vi "Manage Frame.vi"(8 "entrée d'erreur (pas d'erreur)":errorcluster, 10 "Frame Read":string, 11 "Wait_Frame_ERP1 en entrée":refnum<class "Wait_Frame_ERP1.lvclass">) -> (0 "sortie d'erreur":errorcluster, 2 "Frame Ok":bool, 3 "Wait_Frame_ERP1 en sortie":refnum<class "Wait_Frame_ERP1.lvclass">)   [LabVIEW 2020, in "Library Test.lvlib" / "Wait_Frame_ERP1.lvclass"]
uses:
  Wait_Frame_ERP1.lvclass
  UART/UART Enocean/Parsing Data Enocean (Default)/Parsing Data Enocean (Default).lvclass
  C:/Users/ngarcin/OneDrive - Altyor/Standard TB/Suite TB45/Class/UART/UART (Default)/Parsing Data (Default)/Parsing Data (Default).lvclass
  Wait_Frame_ERP1.lvclass/Wait_Frame_ERP1.ctl
  Commun VI/TypeDef/Variable Printable.ctl
  UART/UART Enocean/Parsing Data RADIO_ERP1_A5/Parsing Data RADIO_ERP1_A5.lvclass
  C:/Users/ngarcin/OneDrive - Altyor/Standard TB/Suite TB45/Class/UART/UART Enocean/Parsing Data RADIO_ERP1/Parsing Data RADIO_ERP1.lvclass
  UART/UART Enocean/Parsing Data RADIO_ERP1_A5_H/Parsing Data RADIO_ERP1_A5_H.lvclass
  UART/UART Enocean/Parsing Data RADIO_ERP1_D5/Parsing Data RADIO_ERP1_D5.lvclass
  Commun VI/Library Commun.lvlib
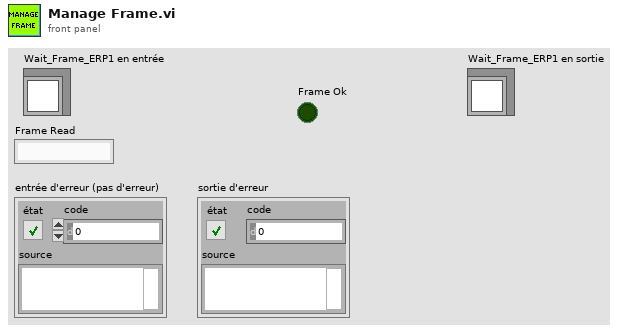
[diagram p1: front panel]
types:
  T1 = typedef "Variable Printable.ctl" = string
  T2 = enum16{"Get Variable", "Get All Variables", "Set Variable", "Delete Variable", "Delete All Variable"}
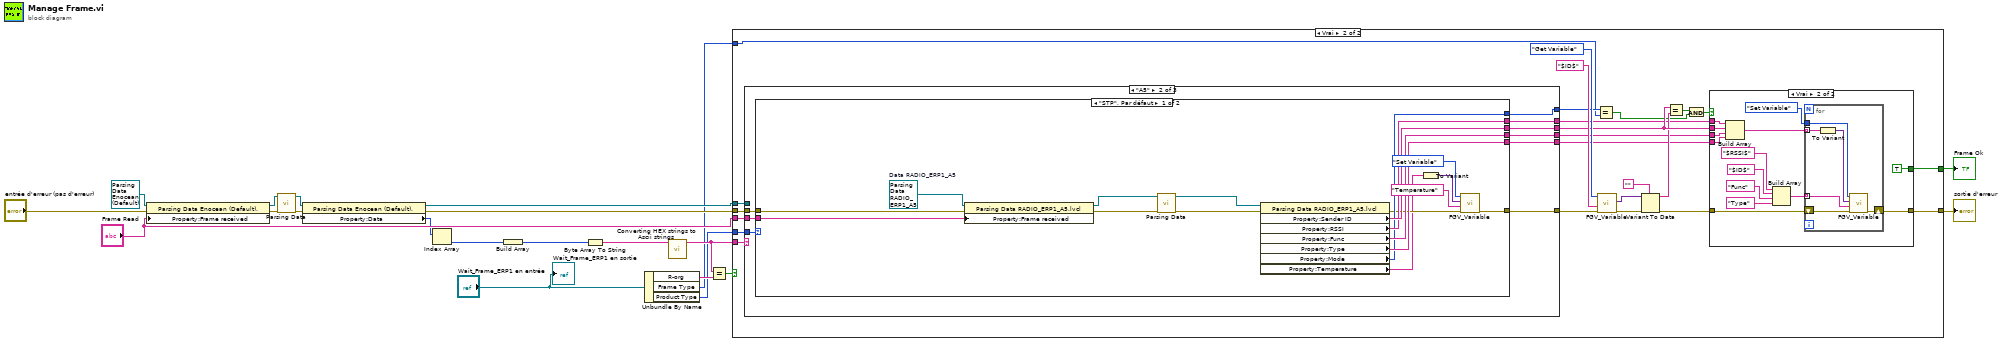
[diagram p0: block diagram]
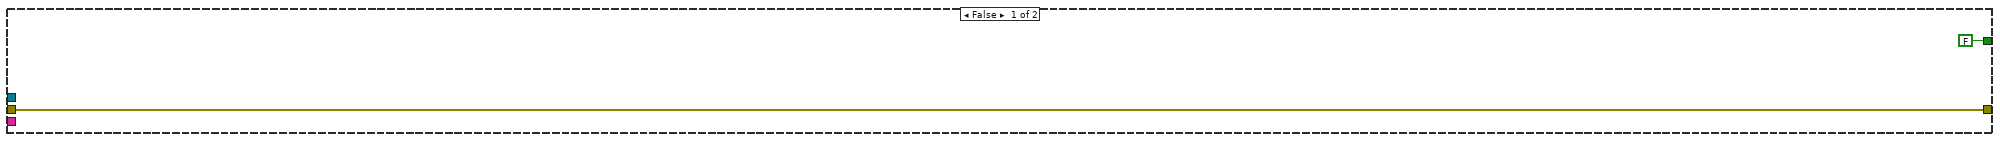
[diagram p2: hidden frame]
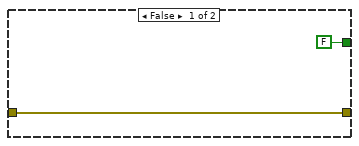
[diagram p3: hidden frame]
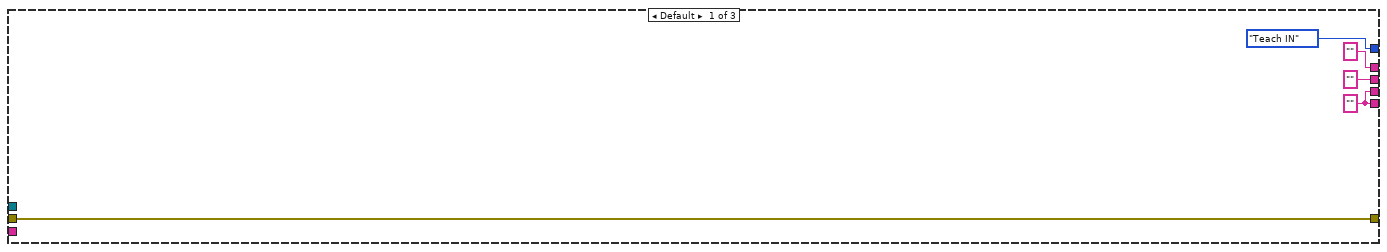
[diagram p4: hidden frame]
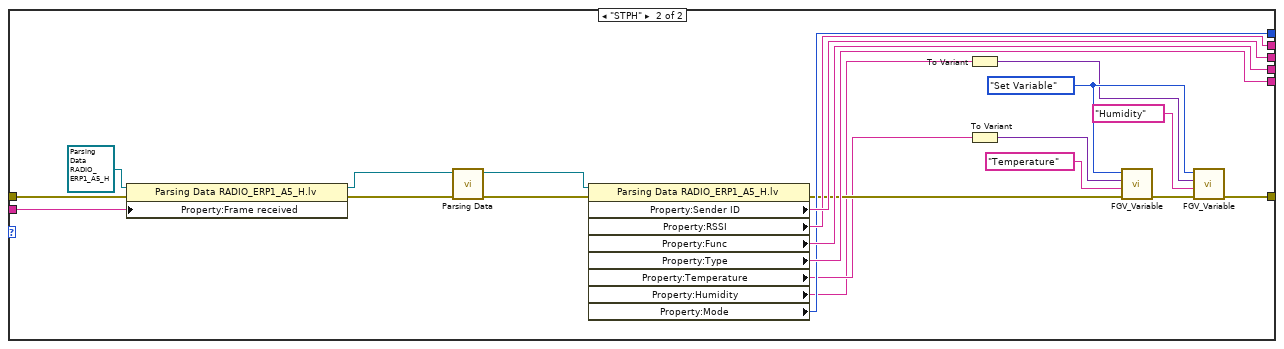
[diagram p5: hidden frame]
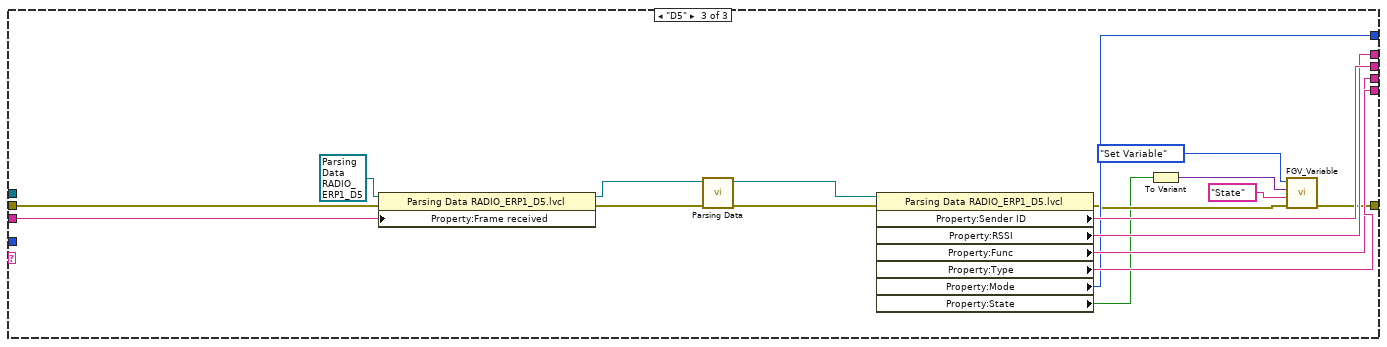
[diagram p6: hidden frame]
diagram:
  n1 = property class="Parsing Data Enocean (Default)."(reference=refnum<class "Parsing Data Enocean (Default).lvclass"> refnum ("Library UART.lvlib:Parsing Data Enocean (Default).lvclass"), error in="entrée d'erreur (pas d'erreur)", "Property:Frame received"="Frame Read") -> (reference out=w14:refnum<class "Parsing Data Enocean (Default).lvclass">, error out=w15:errorcluster)
  n2 = call-dynamic "Parsing Data.vi"("error in (no error)"=w15, "Parsing Enocean (Default) en entrée"=w14) -> ("error out"=w11:errorcluster, "Parsing Enocean (Default) en sortie"=w13:refnum<class "Parsing Data Enocean (Default).lvclass">)  [unwired: 8 in]
  n3 = property class="Parsing Data Enocean (Default)."(reference=w13, error in=w11) -> (reference out=w9:refnum<class "Parsing Data Enocean (Default).lvclass">, error out=w10:errorcluster, "Property:Data"=w12:u8[])
  n4 = Index Array(array=w12) -> (element=w17:u8)  [unwired: 1 in]
  n5 = Build Array(w17) -> (w16:u8[])
  n6 = Byte Array To String(unsigned byte array=w16) -> (string=w18:string)
  n7 = Unbundle By Name("Wait_Frame_ERP1 en entrée") -> ("R-org"=w5:string, "Frame Type"=w2:enum16{"Teach IN", "Normal Mode"}, "Product Type"=w1:enum16{"STP", "STPH", "SDO"})
  n8 = call "Converting HEX strings to Ascii strings.vi"("chaîne IN"=w18) -> ("Chaîne OUT"=w6:string)  [unwired: 9 in, 1 out]
  n9 = Equal?(x=w6, y=w5) -> (x = y?=w4:bool)
  n10 = case shown="Vrai" w4 {
    tunnel: "Frame Read" -> [_ w47]
    tunnel: w10 -> [w23 w46]
    tunnel: w9 -> [_ w45]
    tunnel: [w23 w44] -> w7
    tunnel: w6 -> [_ w43]
    tunnel: [FALSE w33] -> w3
    tunnel: w2 -> [_ w28]
    tunnel: w1 -> [_ w24]
    frame False {
    }
    frame True {
      n11 = case shown="\"A5\"" w43 {
        tunnel: w46 -> [w74 w82 w137]
        tunnel: w45 -> [_ _ _]
        tunnel: [w74 w83 w126] -> w38
        tunnel: [w71 w78 w131] -> w31
        tunnel: ["" ("Property:Sender ID") w81 w135] -> w35
        tunnel: ["" ("Property:RSSI") w79 w134] -> w32
        tunnel: w47 -> [_ w80 w133]
        tunnel: [w71 w77 w132] -> w30
        tunnel: [enum16{"Teach IN", "Normal Mode"}."Teach IN" ("Property:Mode") w76 w130] -> w29
        tunnel: w24 -> [_ w75 _]
        frame Default {
          w71 = "" ("Property:Temperature")
        }
        frame "A5" {
          n12 = case shown="\"STP\", Par défaut" w75 {
            tunnel: [w86 w105] -> w83
            tunnel: w82 -> [w97 w119]
            tunnel: [w96 w118] -> w81
            tunnel: w80 -> [w95 w117]
            tunnel: [w93 w116] -> w79
            tunnel: [w92 w115] -> w78
            tunnel: [w91 w114] -> w77
            tunnel: [w90 w113] -> w76
            frame "STP", Default {
              w94 = refnum<class "Parsing Data RADIO_ERP1_A5.lvclass"> refnum  # Data RADIO_ERP1_A5
              n13 = property class="Parsing Data RADIO_ERP1_A5.lvcl"(reference=w94, error in=w97, "Property:Frame received"=w95) -> (reference out=w99:refnum<class "Parsing Data RADIO_ERP1_A5.lvclass">, error out=w98:errorcluster)
              n14 = call-dynamic "Parsing Data.vi"("error in (no error)"=w98, "Parsing Data RADIO_ERP1 en entrée"=w99) -> ("error out"=w101:errorcluster, "Parsing Data RADIO_ERP1 en sortie"=w100:refnum<class "Parsing Data RADIO_ERP1_A5.lvclass">)  [unwired: 8 in]
              n15 = property class="Parsing Data RADIO_ERP1_A5.lvcl"(reference=w100, error in=w101) -> (error out=w87:errorcluster, "Property:Sender ID"=w96:string, "Property:RSSI"=w93:string, "Property:Func"=w92:string, "Property:Type"=w91:string, "Property:Mode"=w90:enum16{"Teach IN", "Normal Mode"}, "Property:Temperature"=w84:string)  [unwired: 1 out]
              n16 = To Variant(anything=w84) -> (Variant=w89:variant)
              n17 = call "FGV_Variable.vi"("error in (no error)"=w87, "Variable"=T1 "Temperature", "Data In"=w89, "Function"=T2."Set Variable") -> ("error out"=w86:errorcluster)  [unwired: 5 in, 2 out]
            }
            frame "STPH" {
              w107 = T2."Set Variable" ("Function")
              n18 = property class="Parsing Data RADIO_ERP1_A5_H.lv"(reference=refnum<class "Parsing Data RADIO_ERP1_A5_H.lvclass"> refnum ("Library UART.lvlib:Parsing Data RADIO_ERP1_A5_H.lvclass"), error in=w119, "Property:Frame received"=w117) -> (reference out=w121:refnum<class "Parsing Data RADIO_ERP1_A5_H.lvclass">, error out=w120:errorcluster)
              n19 = call-dynamic "Parsing Data.vi"("error in (no error)"=w120, "Parsing Data RADIO_ERP1 en entrée"=w121) -> ("error out"=w123:errorcluster, "Parsing Data RADIO_ERP1 en sortie"=w122:refnum<class "Parsing Data RADIO_ERP1_A5_H.lvclass">)  [unwired: 8 in]
              n20 = property class="Parsing Data RADIO_ERP1_A5_H.lv"(reference=w122, error in=w123) -> (error out=w111:errorcluster, "Property:Sender ID"=w118:string, "Property:RSSI"=w116:string, "Property:Func"=w115:string, "Property:Type"=w114:string, "Property:Temperature"=w109:string, "Property:Humidity"=w102:string, "Property:Mode"=w113:enum16{"Teach IN", "Normal Mode"})  [unwired: 1 out]
              n21 = To Variant(anything=w102) -> (Variant=w103:variant)
              n22 = To Variant(anything=w109) -> (Variant=w110:variant)
              n23 = call "FGV_Variable.vi"("error in (no error)"=w111, "Variable"=T1 "Temperature", "Data In"=w110, "Function"=w107) -> ("error out"=w106:errorcluster)  [unwired: 5 in, 2 out]
              n24 = call "FGV_Variable.vi"("error in (no error)"=w106, "Variable"=T1 "Humidity", "Data In"=w103, "Function"=w107) -> ("error out"=w105:errorcluster)  [unwired: 5 in, 2 out]
            }
          }
        }
        frame "D5" {
          n25 = property class="Parsing Data RADIO_ERP1_D5.lvcl"(reference=refnum<class "Parsing Data RADIO_ERP1_D5.lvclass"> refnum ("Library UART.lvlib:Parsing Data RADIO_ERP1_D5.lvclass"), error in=w137, "Property:Frame received"=w133) -> (reference out=w139:refnum<class "Parsing Data RADIO_ERP1_D5.lvclass">, error out=w138:errorcluster)
          n26 = call-dynamic "Parsing Data.vi"("error in (no error)"=w138, "Parsing Data RADIO_ERP1 en entrée"=w139) -> ("error out"=w141:errorcluster, "Parsing Data RADIO_ERP1 en sortie"=w140:refnum<class "Parsing Data RADIO_ERP1_D5.lvclass">)  [unwired: 8 in]
          n27 = property class="Parsing Data RADIO_ERP1_D5.lvcl"(reference=w140, error in=w141) -> (error out=w127:errorcluster, "Property:Sender ID"=w135:string, "Property:RSSI"=w134:string, "Property:Func"=w131:string, "Property:Type"=w132:string, "Property:Mode"=w130:enum16{"Teach IN", "Normal Mode"}, "Property:State"=w125:bool)  [unwired: 1 out]
          n28 = To Variant(anything=w125) -> (Variant=w129:variant)
          n29 = call "FGV_Variable.vi"("error in (no error)"=w127, "Variable"=T1 "State", "Data In"=w129, "Function"=T2."Set Variable") -> ("error out"=w126:errorcluster)  [unwired: 5 in, 2 out]
        }
      }
      n30 = Equal?(x=w29, y=w28) -> (x = y?=w25:bool)
      n31 = call "FGV_Variable.vi"("error in (no error)"=w38, "Variable"=T1 "$ID$", "Function"=T2."Get Variable") -> ("error out"=w40:errorcluster, "Data Out"=w37:variant)  [unwired: 6 in, 1 out]
      n32 = Variant To Data(error in=w40, type="", Variant=w37) -> (data=w34:string, error out=w36:errorcluster)
      n33 = Equal?(x=w35, y=w34) -> (x = y?=w27:bool)
      n34 = And(x=w27, y=w25) -> (x .and. y?=w26:bool)
      n35 = case shown="Vrai" w26 {
        tunnel: [w49 w54] -> w44
        tunnel: w36 -> [w49 w62]
        tunnel: w35 -> [_ w56]
        tunnel: [FALSE TRUE] -> w33
        tunnel: w32 -> [_ w57]
        tunnel: w31 -> [_ w51]
        tunnel: w30 -> [_ w50]
        frame False {
        }
        frame True {
          n36 = Build Array(w57, w56, w51, w50) -> (w55:string[])
          n37 = Build Array(T1 "$RSSI$" ("Variable"), T1 "$ID$" ("Variable"), T1 "Func" ("Variable"), T1 "Type" ("Variable")) -> (w58:T1[])
          n38 = for {
            tunnel: w58 -> [w69] mode=indexing
            tunnel: T2."Set Variable" ("Function") -> [w68]
            shift-right: [w67] -> w54
            shift-left: w62 -> [w66]
            tunnel: w55 -> [w65] mode=indexing
            n39 = To Variant(anything=w65) -> (Variant=w64:variant)
            n40 = call "FGV_Variable.vi"("error in (no error)"=w66, "Variable"=w69, "Data In"=w64, "Function"=w68) -> ("error out"=w67:errorcluster)  [unwired: 5 in, 2 out]
          }
        }
      }
    }
  }
  "sortie d'erreur" <- w7
  "Frame Ok" <- w3
  "Wait_Frame_ERP1 en sortie" <- "Wait_Frame_ERP1 en entrée"
